vi "Create Channels from Parameter List (BC).vi"(7 "Message Param map in":T1, 8 "error in (no error)":errorcluster, 10 "Param ID map in":map{i32, string}(c390), 11 "channel ref in":T6=18446744073709551615 format="%.0x") -> (0 "error out":errorcluster, 2 "Param ID map out":map{i32, string}(c390), 3 "channel ref out":T6=18446744073709551615 format="%.0x", 5 "Message Param map out":T1)   [LabVIEW 2020, in "Ballard 1553 System Explorer.lvlib"]
uses:
  Ballard 1553 System Explorer.lvlib
  <vilib>/NI VeriStand/Custom Device API/Custom Device Item Ref.ctl
  param_sysdef_type.ctl
  param_map_sysdef_type.ctl
  Shared/Configuration/_typedefs/param_type.ctl
  Shared/Configuration/_typedefs/param_signalType_type.ctl
  Shared/Configuration/_typedefs/param_encoding_type.ctl
  Parse XML Ballard/Ballard_messageType.ctl
  <vilib>/NI VeriStand/Custom Device API/Custom Device Channel Type.ctl
  Shared/Controls and Global/Global.vi
  <vilib>/NI VeriStand/Custom Device Tools/Custom Device Utility Library/NI VeriStand - Search for Item by GUID.vi
  <vilib>/NI VeriStand/Custom Device Tools/Custom Device Utility Library/NI VeriStand - Search for All Items by GUID.vi
  <vilib>/NI VeriStand/Custom Device API/Get Item Property (I32).vi
  <vilib>/NI VeriStand/Custom Device API/Get Item Property (U16).vi
  <vilib>/NI VeriStand/Custom Device Tools/Custom Device Utility Library/Custom Device Utility Library.lvlib
  Shared/Ballard 1553 Shared.lvlib
  <vilib>/NI VeriStand/Custom Device API/Custom Device API.lvlib
  Shared/Configuration/Configuration_Helper.lvlib
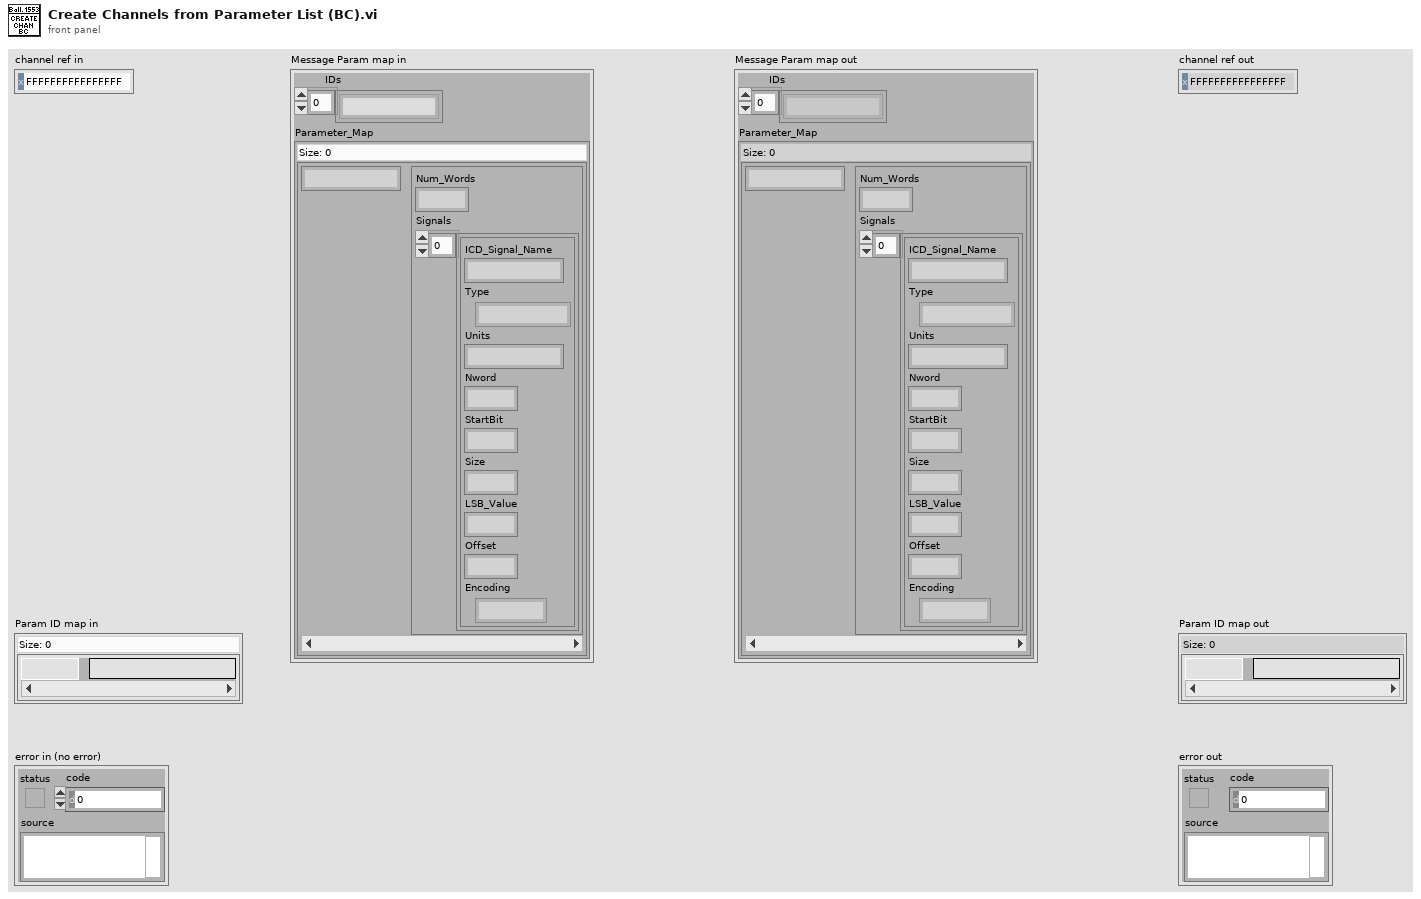
[diagram p1: front panel]
types:
  T1 = typedef "Ballard 1553 System Explorer.lvlib/param_sysdef_type.ctl" = cluster{"IDs":string[], "Parameter_Map":map{string, T2}}
  T2 = typedef "Ballard 1553 System Explorer.lvlib/param_map_sysdef_type.ctl" = cluster{"Num_Words":u8, "Signals":T3[]}
  T3 = typedef "Configuration_Helper.lvlib/param_type.ctl" = cluster{"ICD_Signal_Name":string, "Type":T4, "Units":string, "Nword":i32, "StartBit":i32, "Size":i32, "LSB_Value":dbl, "Offset":i32, "Encoding":T5}
  T4 = typedef "Configuration_Helper.lvlib/param_signalType_type.ctl" = enum16{"Opaque", "Enum", "Float", "Integer", "Bcd", "Bool"}
  T5 = typedef "Configuration_Helper.lvlib/param_encoding_type.ctl" = enum16{"None", "2-complement", "Unsigned"}
  T6 = typedef "Custom Device API.lvlib/Custom Device Item Ref.ctl" = u64
  T7 = typedef "Ballard 1553 System Explorer.lvlib/Ballard_messageType.ctl" = enum16{"BC to RT", "RT to BC", "RT to RT", "MC (Rx)", "MC (Tx)"}
  T8 = typedef "Custom Device API.lvlib/Custom Device Channel Type.ctl" = enum16{"Input", "Output"}
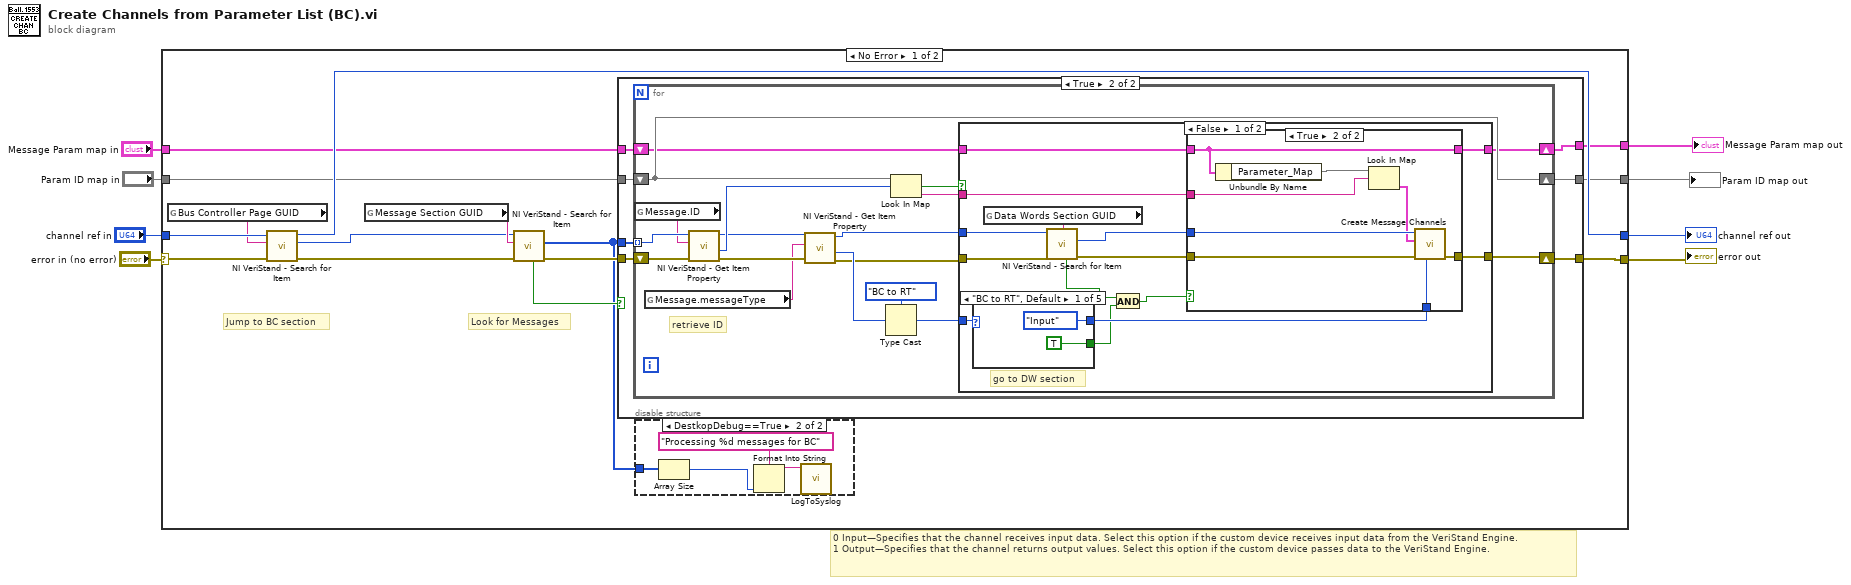
[diagram p0: block diagram]
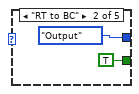
[diagram p4: hidden frame]
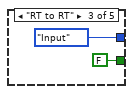
[diagram p5: hidden frame]
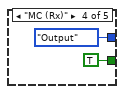
[diagram p6: hidden frame]
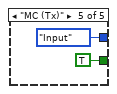
[diagram p7: hidden frame]
diagram:
  # "0 Input—Specifies that the channel receives input data. Select this option if the custom device receives input data from the VeriStand Engine. \n1 Output—Specifies that the channel returns output values. Select this option if the custom device passes data to the VeriStand Engine."
  n1 = case shown="No Error" "error in (no error)" {
    selector: "error in (no error)" -> [w22 w93]
    tunnel: "channel ref in" -> [w23 w95]
    tunnel: "Param ID map in" -> [w14 w94]
    tunnel: [w21 w95] -> w5
    tunnel: [w13 w94] -> w4
    tunnel: [w17 w93] -> w3
    tunnel: "Message Param map in" -> [w12 w92]
    tunnel: [w11 w92] -> w1
    frame No Error {
      # "Look for Messages"
      # "Jump to BC section"
      n2 = global read "Global.vi" "Bus Controller Page GUID"() -> (w10:string)
      n3 = call-poly <vilib>:"NI VeriStand - Search for Item.vi"("error in"=w22, "Item GUID"=w10, "Section Ref in"=w23) -> ("error out"=w20:errorcluster, "Item Ref"=w15:T6, "Section Ref out"=w21:T6)  [unwired: 5 in, 1 out]
      n4 = global read "Global.vi" "Message Section GUID"() -> (w19:string)
      n5 = call-poly <vilib>:"NI VeriStand - Search for Item.vi"("error in"=w20, "Item GUID"=w19, "Section Ref in"=w15) -> ("error out"=w16:errorcluster, "Item Refs"=w9:T6[], "Found"=w18:bool)  [unwired: 5 in, 1 out]
      n6 = case shown="True" w18 {
        tunnel: w9 -> [_ w37]
        tunnel: [w30 w35] -> w17
        tunnel: w16 -> [w30 w36]
        tunnel: w14 -> [w29 w34]
        tunnel: [w29 w33] -> w13
        tunnel: w12 -> [w28 w32]
        tunnel: [w28 w31] -> w11
        frame False {
        }
        frame True {
          n7 = for {
            tunnel: w37 -> [w53] mode=indexing
            shift-right: [w55] -> w35
            shift-left: w36 -> [w54]
            shift-right: [w51] -> w33
            shift-left: w34 -> [w51]
            shift-right: [w46] -> w31
            shift-left: w32 -> [w47]
            # "retrieve ID"
            n8 = global read "Global.vi" "Message.ID"() -> (w52:string)
            n9 = global read "Global.vi" "Message.messageType"() -> (w43:string)
            n10 = call-poly <vilib>:"NI VeriStand - Get Item Property.vi"("error in (no error)"=w54, "Property Name"=w52, "Item Ref in"=w53) -> ("error out"=w44:errorcluster, "Value"=w50:i32, "Item Ref out"=w45:T6)  [unwired: 5 in, 1 out]
            n11 = call-poly <vilib>:"NI VeriStand - Get Item Property.vi"("error in (no error)"=w44, "Property Name"=w43, "Item Ref in"=w45) -> ("error out"=w40:errorcluster, "Value"=w41:u16, "Item Ref out"=w39:T6)  [unwired: 5 in, 1 out]
            n12 = Type Cast(type=Ballard_messageType."BC to RT" ("messageType"), x=w41) -> (*(type *) &x=w38:T7)
            n13 = Look In Map(map=w51, key=w50) -> (key not found?=w49:bool, value=w48:string)  [unwired: 1 in]
            n14 = case shown="False" w49 {
              tunnel: [w64 w91] -> w55
              tunnel: w39 -> [w69 _]
              tunnel: w40 -> [w68 w91]
              tunnel: w48 -> [w58 _]
              tunnel: w47 -> [w63 w90]
              tunnel: [w62 w90] -> w46
              tunnel: w38 -> [w59 _]
              frame False {
                # "go to DW section"
                n15 = case shown="\"BC to RT\", Default" w59 {
                  tunnel: [Custom_Device_Channel_Type."Input" ("VS channel direction") Custom_Device_Channel_Type."Output" ("VS channel direction") Custom_Device_Channel_Type."Input" ("VS channel direction") Custom_Device_Channel_Type."Output" ("VS channel direction") Custom_Device_Channel_Type."Input" ("VS channel direction")] -> w60
                  tunnel: [TRUE TRUE FALSE TRUE TRUE] -> w56
                  frame "BC to RT", Default {
                  }
                  frame "RT to BC" {
                  }
                  frame "RT to RT" {
                  }
                  frame "MC (Rx)" {
                  }
                  frame "MC (Tx)" {
                  }
                }
                n16 = global read "Global.vi" "Data Words Section GUID"() -> (w61:string)
                n17 = call-poly <vilib>:"NI VeriStand - Search for Item.vi"("error in"=w68, "Item GUID"=w61, "Section Ref in"=w69) -> ("error out"=w67:errorcluster, "Item Ref"=w66:T6, "Found"=w65:bool)  [unwired: 5 in, 1 out]
                n18 = And(x=w65, y=w56) -> (x .and. y?=w57:bool)
                n19 = case shown="True" w57 {
                  tunnel: w67 -> [w80 w89]
                  tunnel: w66 -> [_ w88]
                  tunnel: [w80 w87] -> w64
                  tunnel: w63 -> [w81 w84]
                  tunnel: [w81 w84] -> w62
                  tunnel: w60 -> [_ w86]
                  tunnel: w58 -> [_ w85]
                  frame False {
                  }
                  frame True {
                    n20 = Unbundle By Name(w84) -> ("Parameter_Map"=w83:map{string, T2})
                    n21 = Look In Map(map=w83, key=w85) -> (value=w82:T2)  [unwired: 1 in, 1 out]
                    n22 = call "Create Message Channels.vi"("VS channel direction"=w86, "error in (no error)"=w89, "Parameters"=w82, "Data Words section in"=w88) -> ("error out"=w87:errorcluster)  [unwired: 6 in, 1 out]
                  }
                }
              }
              frame True {
              }
            }
          }
        }
      }
      n23 = disable-structure shown="DestkopDebug==True" {
        disable-tunnel: w9 -> [_ w26]
        frame condition #0 {
        }
        frame condition #1 (active) {
          n24 = Array Size(array=w26) -> (size(s)=w25:i32)
          n25 = Format Into String(format string="Processing %d messages for BC", w25) -> (resulting string=w24:string)  [unwired: 2 in, 1 out]
          n26 = call "LogToSyslog.vi"("message"=w24) -> ()  [unwired: 9 in, 2 out]
        }
      }
    }
    frame Error {
    }
  }
  "error out" <- w3
  "channel ref out" <- w5
  "Param ID map out" <- w4
  "Message Param map out" <- w1
